vi "Test.Mathematica.vi"() -> ()   [LabVIEW 2014]
panel:
  out "Now (us)":dbl=1.0 format="%.2f"
  in  "Parameter":u16(ring) items=["Frequency (MHz)", "Amplitude (dBm)", "Phase (Pi)"]
  in  "Start":i32=1
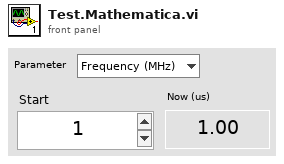
[diagram p1: front panel]
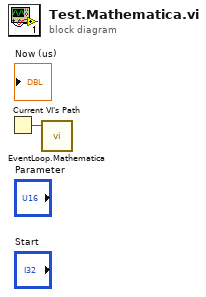
[diagram p0: block diagram]
diagram:
  n1 = Current VI's Path() -> (path=w1:path)
  n2 = call "EventLoop.Mathematica.vi"("Path"=w1) -> ()  [unwired: 2 in]
